vi "query.vi"(8 "error in (no error)":errorcluster, 10 "condition":string, 11 "database in":refnum<class "database.lvclass">) -> (0 "error out":errorcluster, 1 "data":variant[][](array[variant]), 3 "database out":refnum<class "database.lvclass">)   [LabVIEW 2018, in "database.lvclass"]
uses:
  database.lvclass
  database.lvclass/database.ctl
  <vilib>/addons/database/NI_Database_API.lvlib
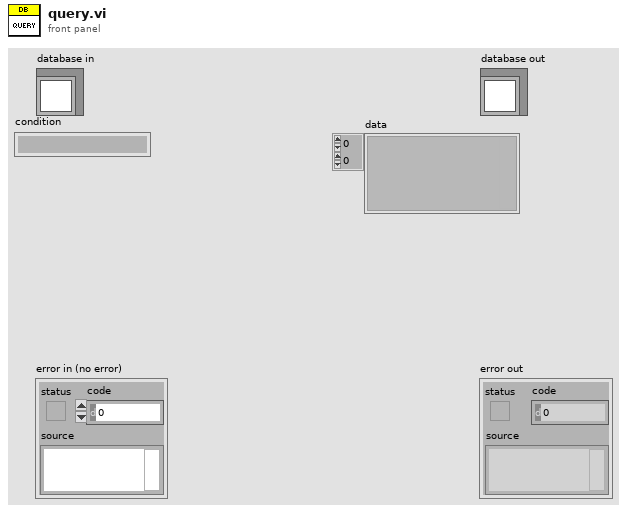
[diagram p1: front panel]
types:
  T1 = typedef "NI_Database_API.lvlib/Conn ObjectReference.ctl" = refnum<k1>
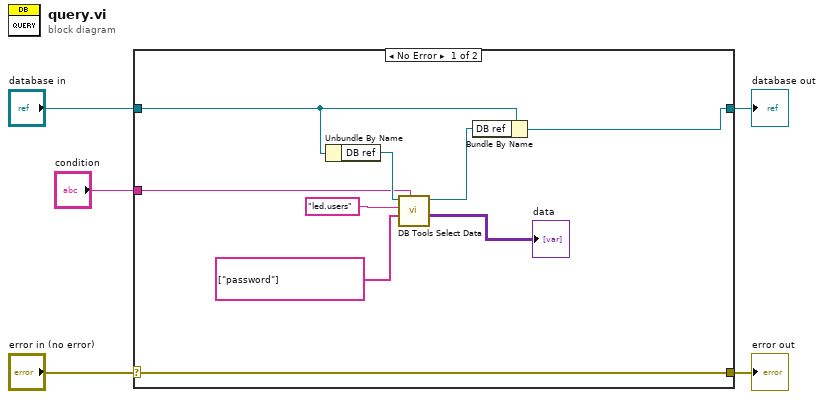
[diagram p0: block diagram]
diagram:
  n1 = case shown="No Error" "error in (no error)" {
    selector: "error in (no error)" -> [w14 w16]
    tunnel: [w14 w16] -> w4
    tunnel: [w9 w15] -> w2
    tunnel: "database in" -> [w10 w15]
    tunnel: "condition" -> [w11 _]
    frame No Error {
      n2 = Unbundle By Name(w10) -> ("DB ref"=w13:T1)
      n3 = call <vilib>:"DB Tools Select Data.vi"("condition"=w11, "columns"=string[] ["password"], "table"="led.users", "connection reference"=w13) -> ("data"=→"data":variant[][], "connection reference out"=w8:T1)  [unwired: 2 in, 1 out]
      n4 = Bundle By Name(cluster=w10, "DB ref"=w8) -> (w9:refnum<class "database.lvclass">)
    }
    frame Error {
    }
  }
  "error out" <- w4
  "database out" <- w2
